vi "DefaultFromIni.vi"(8 "error in (no error)":errorcluster, 11 "SamplerPluginsBase in":refnum<class "SamplerPluginsBase.lvclass">) -> (0 "error out":errorcluster, 3 "SamplerPluginsBase out":refnum<class "SamplerPluginsBase.lvclass">)   [LabVIEW 2014, in "SamplerPlugins.lvlib" / "SamplerPluginsBase.lvclass"]
uses:
  SamplerPluginsBase.lvclass
  <vilib>/Utility/config.llb/NI_LVConfig.lvlib
  <vilib>/Utility/error.llb/Error Cluster From Error Code.vi
  <vilib>/ErrorRing/Error Ring.xnode
  TypeDefs/CorrectionFactors.ctl
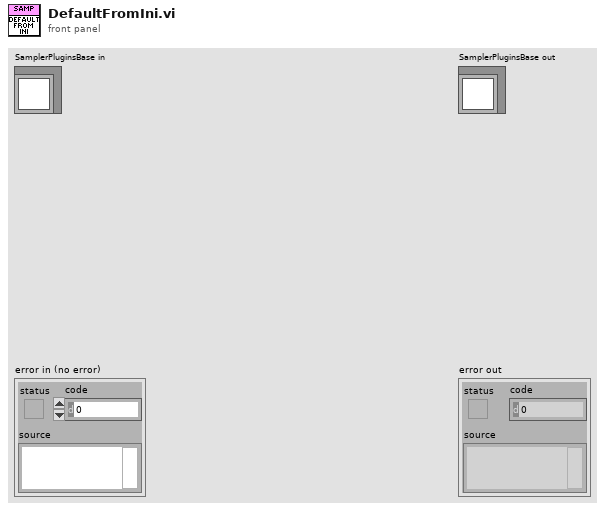
[diagram p1: front panel]
types:
  T1 = typedef "SamplerPlugins.lvlib/SamplerPluginsBase.lvclass/CorrectionFactors.ctl" = cluster{"MagCorr":dbl[], "DlyCorr":dbl[]}
  T2 = typedef "SamplerPlugins.lvlib/SamplerPluginsBase.lvclass/DefaultINIParams.ctl" = cluster{"Handle":string, "eFunction":u16, "dRange":dbl, "dResolution":dbl, "eTriggerSource":u16, "dTriggerDelay":dbl, "iMaxTimeMilliseconds":i32, "eMeasCompleteDest":u16, "iTriggerCount":i32, "iSampleCount":i32, "eSampleClock":u16, "dSampleInterval":dbl, "iMaxTimeMillisecondsMultiPoint":i32, "iArraySize":i32, "dMinFreq":dbl, "dMaxFreq":dbl, "dFrequencyVoltageRange":dbl, "eEdge":u16, "sSource":string, "eEdgeSample":u16, "sSourceSample":string}
  T3 = typedef "NI_LVConfig.lvlib/Config Data RefNum.ctl" = refnum<k1>
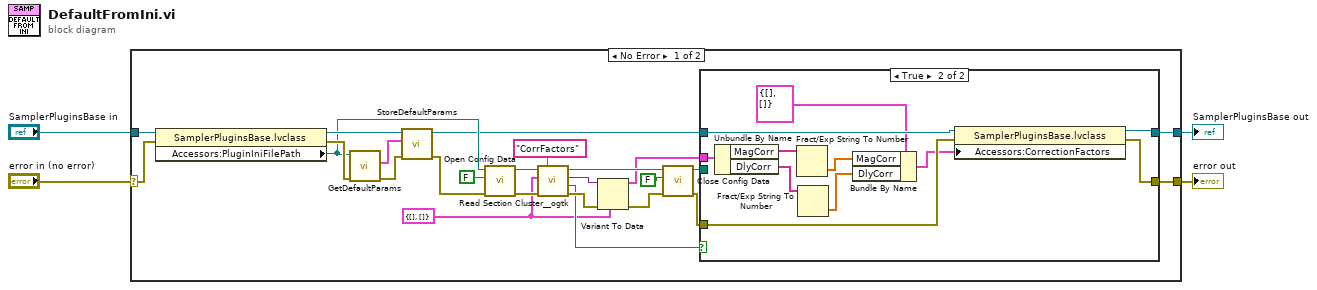
[diagram p0: block diagram]
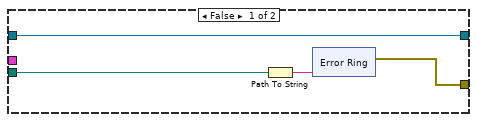
[diagram p2: hidden frame]
diagram:
  n1 = case shown="No Error" "error in (no error)" {
    selector: "error in (no error)" -> [w28 w53]
    tunnel: [w14 w53] -> w3
    tunnel: [w8 w52] -> w1
    tunnel: "SamplerPluginsBase in" -> [w29 w52]
    frame No Error {
      w15 = cluster{"MagCorr":string[], "DlyCorr":string[]} {"MagCorr"=[], "DlyCorr"=[]} ("CorrectionFactors")
      n2 = property class="SamplerPluginsBase.lvclass"(reference=w29, error in=w28) -> (reference out=w26:refnum<class "SamplerPluginsBase.lvclass">, error out=w27:errorcluster, "Accessors:PluginIniFilePath"=w21:path)
      n3 = call "GetDefaultParams.vi"("error in (no error)"=w27, "config file path"=w21) -> ("error out"=w24:errorcluster, "DefaultINIParams"=w25:T2)  [unwired: 8 in]
      n4 = call "StoreDefaultParams.vi"("error in (no error)"=w24, "DefaultINIParams"=w25, "NISTSamplerPluginsBase in"=w26) -> ("error out"=w22:errorcluster, "NISTSamplerPluginsBase out"=w10:refnum<class "SamplerPluginsBase.lvclass">)  [unwired: 7 in]
      n5 = call <vilib>:"Open Config Data.vi"("error in (no error)"=w22, "create file if necessary (T)"=FALSE, "configuration file path"=w21) -> ("error out"=w20:errorcluster, "refnum"=w19:T3)  [unwired: 6 in, 1 out]
      n6 = call <userlib>:"Read Section Cluster__ogtk.vi"("section (optional)"="CorrFactors", "error in (no error)"=w20, "Section Formatted Cluster Type"=w15, "refnum"=w19) -> ("error out"=w18:errorcluster, "all found?"=w16:bool, "Section Formatted Cluster"=w17:variant, "dup refnum"=w13:T3)  [unwired: 3 in, 1 out]
      n7 = Variant To Data(error in=w18, type=w15, Variant=w17) -> (data=w5:cluster{"MagCorr":string[], "DlyCorr":string[]}, error out=w9:errorcluster)
      n8 = call <vilib>:"Close Config Data.vi"("error in (no error)"=w9, "write file if changed (T)"=FALSE, "refnum"=w13) -> ("error out"=w7:errorcluster, "file path"=w11:path)  [unwired: 7 in]
      n9 = case shown="True" w16 {
        tunnel: [w32 w50] -> w14
        tunnel: w11 -> [w31 _]
        tunnel: w10 -> [w30 w51]
        tunnel: [w30 w49] -> w8
        tunnel: w7 -> [_ w48]
        tunnel: w5 -> [_ w47]
        frame False {
          n10 = Path To String(path=w31) -> (string=w33:string)
          n11 = xnode "Error Ring"("parameter 0"=w33) -> ("error out"=w32:errorcluster)
        }
        frame True {
          n12 = Unbundle By Name(w47) -> ("MagCorr"=w46:string[], "DlyCorr"=w45:string[])
          n13 = Fract/Exp String To Number(string=w46) -> (number=w43:dbl[])  [unwired: 3 in, 1 out]
          n14 = Fract/Exp String To Number(string=w45) -> (number=w42:dbl[])  [unwired: 3 in, 1 out]
          n15 = Bundle By Name(cluster=T1 {"MagCorr"=[], "DlyCorr"=[]} ("CorrectionFactors"), "MagCorr"=w43, "DlyCorr"=w42) -> (w41:T1)
          n16 = property class="SamplerPluginsBase.lvclass"(reference=w51, error in=w48, "Accessors:CorrectionFactors"=w41) -> (reference out=w49:refnum<class "SamplerPluginsBase.lvclass">, error out=w50:errorcluster)
        }
      }
    }
    frame Error {
    }
  }
  "error out" <- w3
  "SamplerPluginsBase out" <- w1
